vi "FGV Rezepte wechseln.vi"(0 "Rezepte":string, 1 "AK/man":T1, 5 "Rezeptindex":i32, 7 "Diesel":u16(ring) caption="Diesel:" items=["---"], 9 "Gasoline":u16(ring) caption="Gasoline:" items=["---"], 11 "error in (no error)":errorcluster caption="Fehler (Eingang, kein Fehler)", 12 "Natural Gas":u16(ring) caption="Natural Gas:" items=["---"], 13 "Aktion":T2) -> (3 "AK/man":T1, 4 "Rezepte":string[](array[string]), 6 "Rezeptindex":i32, 8 "Diesel":u16, 10 "Gasoline":u16, 14 "Natural Gas":u16, 15 "error out":errorcluster caption="Fehler (Ausgang)")   [LabVIEW 2020, in "FT-IR.lvlib"]
uses:
  FT-IR.lvlib
  Aktion FGV Rezepte wechseln.ctl
  AK-manuell.ctl
  Allgemein/allgemeine Sub-VIs.lvlib
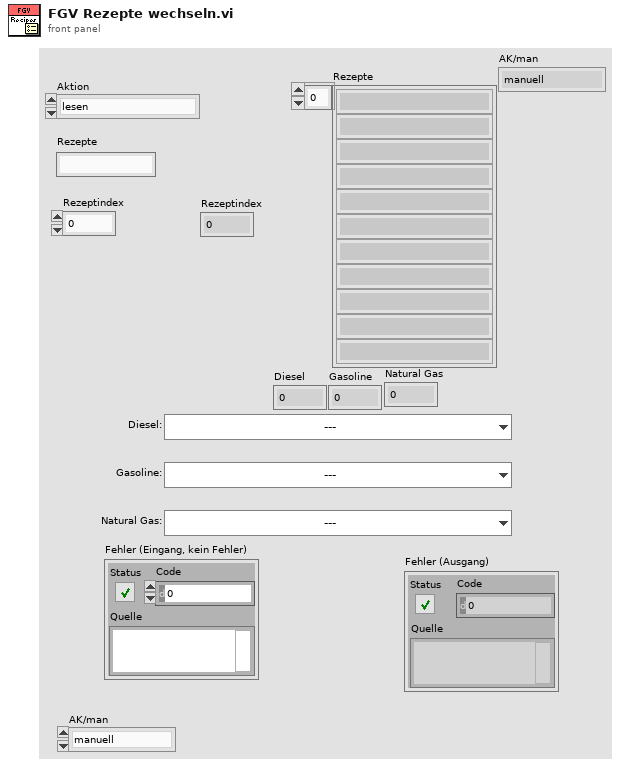
[diagram p1: front panel]
types:
  T1 = typedef "FT-IR.lvlib/AK-manuell.ctl" = enum16{"manuell", "Diesel", "CNG", "Gasoline"}
  T2 = typedef "FT-IR.lvlib/Aktion FGV Rezepte wechseln.ctl" = enum16{"lesen", "Rezepte", "Rezeptindex", "Diesel", "Gasoline", "NCG", "laden", "speichern", "AK/Man"}
  T3 = cluster{"Diesel":u16, "Gasoline":u16, "Natural Gas":u16}
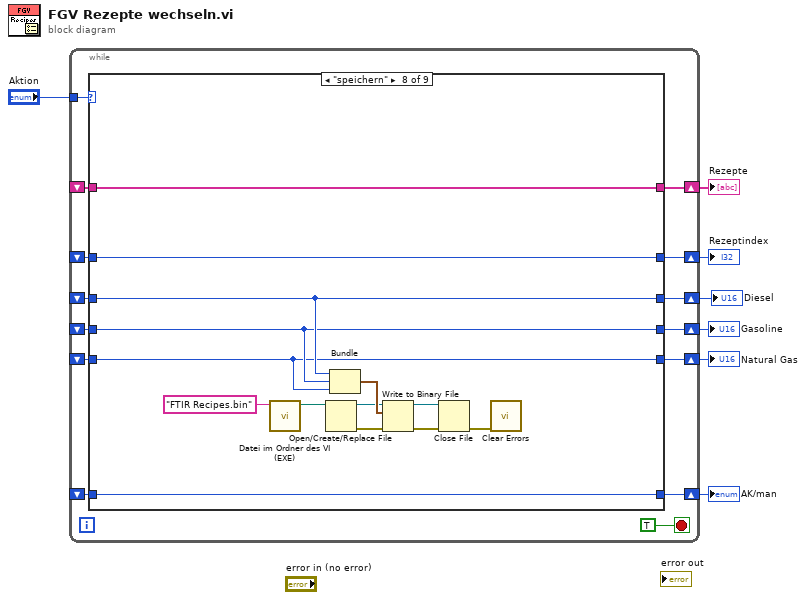
[diagram p0: block diagram]
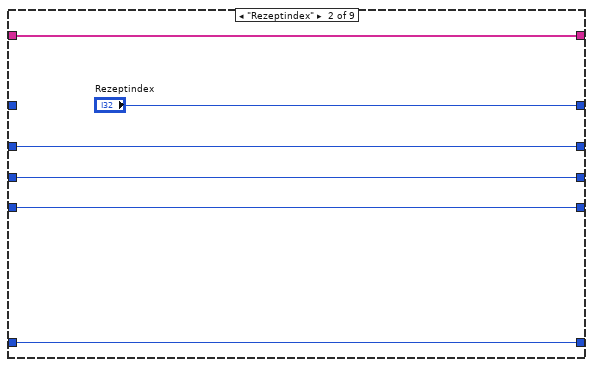
[diagram p3: hidden frame]
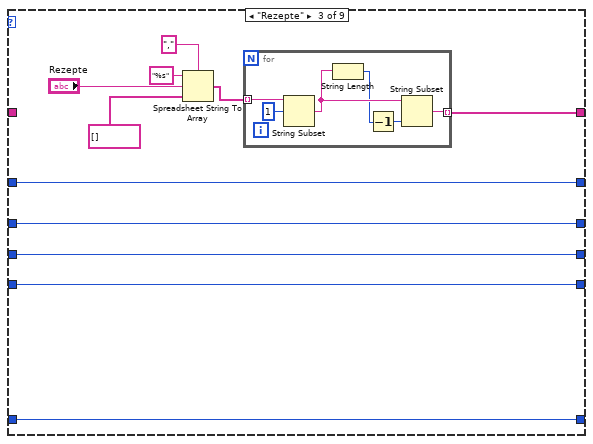
[diagram p4: hidden frame]
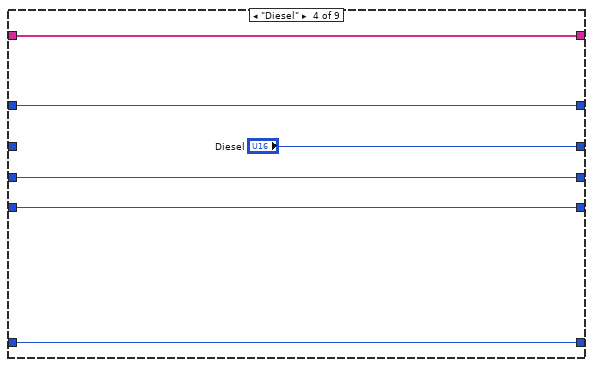
[diagram p5: hidden frame]
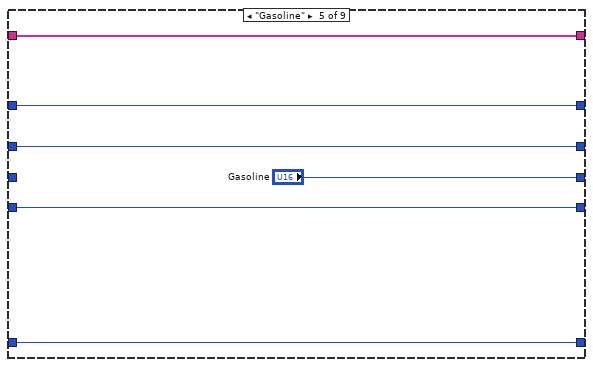
[diagram p6: hidden frame]
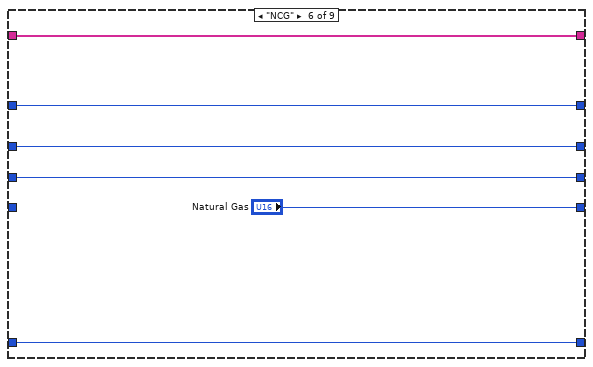
[diagram p7: hidden frame]
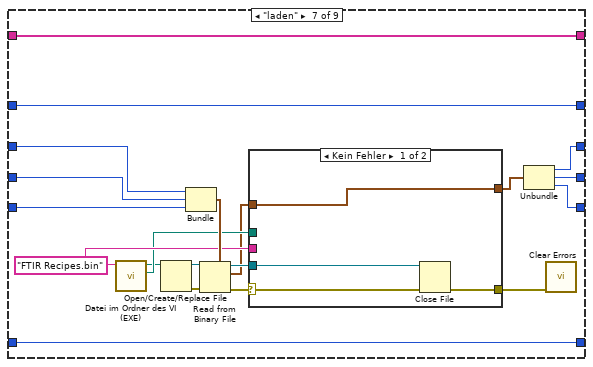
[diagram p8: hidden frame]
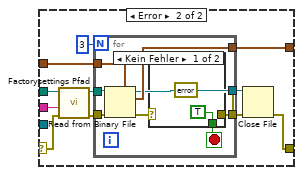
[diagram p9: hidden frame]
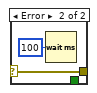
[diagram p10: hidden frame]
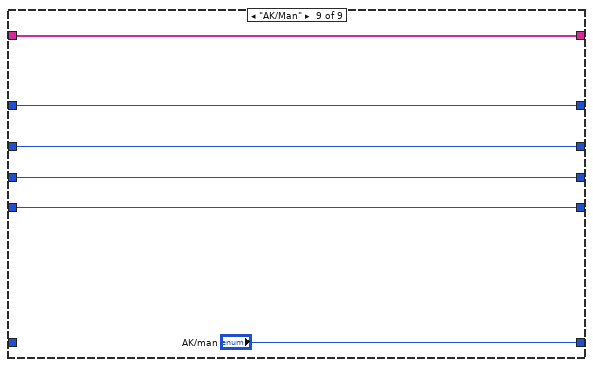
[diagram p11: hidden frame]
diagram:
  n1 = while {
    tunnel: "Aktion" -> [w20]
    shift-right: [w19] -> w6
    shift-left: _ -> [w18]
    shift-right: [w17] -> w5
    shift-left: _ -> [w16]
    shift-right: [w15] -> w4
    shift-left: _ -> [w14]
    shift-right: [w13] -> w3
    shift-left: _ -> [w12]
    shift-right: [w11] -> w2
    shift-left: _ -> [w10]
    shift-right: [w9] -> w1
    shift-left: _ -> [w8]
    stop <- TRUE stop-if-true
    n2 = case shown="\"speichern\"" w20 {
      tunnel: [w27 w33 w39 w56 w62 w68 w88 w129 w135] -> w19
      tunnel: w18 -> [w27 w33 _ w56 w62 w68 w88 w129 w135]
      tunnel: [w26 "Rezeptindex" w38 w55 w61 w67 w87 w128 w134] -> w17
      tunnel: w16 -> [w26 _ w38 w55 w61 w67 w87 w128 w134]
      tunnel: [w25 w31 w37 "Diesel" w60 w66 w82 w126 w133] -> w15
      tunnel: w14 -> [w25 w31 w37 _ w60 w66 w85 w126 w133]
      tunnel: [w24 w30 w36 w53 "Gasoline" w65 w81 w125 w132] -> w13
      tunnel: w12 -> [w24 w30 w36 w53 _ w65 w84 w125 w132]
      tunnel: [w23 w29 w35 w52 w58 "Natural Gas" w80 w124 w131] -> w11
      tunnel: w10 -> [w23 w29 w35 w52 w58 _ w83 w124 w131]
      tunnel: [w22 w28 w34 w51 w57 w63 w79 w122 "AK/man"] -> w9
      tunnel: w8 -> [w22 w28 w34 w51 w57 w63 w79 w122 _]
      frame "lesen", Default {
      }
      frame "Rezeptindex" {
      }
      frame "Rezepte" {
        n3 = Spreadsheet String To Array(delimiter (Tab)="," ("Trennzeichen (Tabulator)"), format string="%s" ("Format-String"), spreadsheet string="Rezepte", array type (2D Dbl)=string[] []) -> (array=w40:string[])
        n4 = for {
          tunnel: w40 -> [w50] mode=indexing
          tunnel: [w45] -> w39 mode=indexing
          n5 = String Subset(string=w50, offset (0)=1 ("Offset (0)")) -> (substring=w48:string)  [unwired: 1 in]
          n6 = String Length(string=w48) -> (length=w46:i32)
          n7 = Decrement(x=w46) -> (x-1=w47:i32)
          n8 = String Subset(string=w48, length (rest)=w47) -> (substring=w45:string)  [unwired: 1 in]
        }
      }
      frame "Diesel" {
      }
      frame "Gasoline" {
      }
      frame "NCG" {
      }
      frame "laden" {
        w76 = "FTIR Recipes.bin" ("Dateiname")
        n9 = call "Datei im Ordner des VI (EXE).vi"("Dateiname"=w76) -> ("Ordner des Haupt-VIs"=w75:path, "Dateipfad im Ordner des Haupt-VIs"=w69:path)  [unwired: 8 in, 1 out]
        n10 = Open/Create/Replace File(file path (use dialog)=w69) -> (refnum out=w70:refnum<file>, error out=w71:errorcluster)  [unwired: 5 in, 1 out]
        n11 = Bundle("Diesel"=w85, "Gasoline"=w84, "Natural Gas"=w83) -> (w86:T3)  [unwired: 1 in]
        n12 = Read from Binary File(5:w86, 8:w71, 11:w70) -> (0:w78:errorcluster, 2:w74:T3, 3:w77:refnum<file>)  [unwired: 4 out]
        n13 = case shown="Kein Fehler" w78 {
          selector: w78 -> [w91 w95]
          tunnel: w75 -> [_ w96]
          tunnel: w74 -> [w92 w94]
          tunnel: [w92 w102] -> w73
          tunnel: [w89 w100] -> w72
          tunnel: w77 -> [w90 _]
          tunnel: w76 -> [_ w93]
          frame No Error {
            n14 = Close File(refnum=w90, error in=w91) -> (error out=w89:errorcluster)  [unwired: 1 out]
          }
          frame Error {
            n15 = call "Factorysettings Pfad.vi"("error in (no error)"=w95, "Dateiname"=w93, "Ordner des Haupt-VIs"=w96) -> ("error out"=w97:errorcluster, "Pfad Factorysettings"=w98:path)  [unwired: 7 in]
            n16 = for {
              N: 3 -> [_]
              tunnel: w97 -> [w109]
              tunnel: w98 -> [w108]
              tunnel: [w107] -> w102
              tunnel: [w106] -> w101
              tunnel: [w105] -> w99
              tunnel: w94 -> [w104]
              stop <- w110 stop-if-true
              n17 = Read from Binary File(5:w104, 8:w109, 11:w108) -> (0:w111:errorcluster, 2:w107:T3, 3:w105:refnum<file>)  [unwired: 3 in, 1 out]
              n18 = case shown="Kein Fehler" w111 {
                selector: w111 -> [_ w114]
                tunnel: [TRUE _] -> w110
                tunnel: [errorcluster {"status"=FALSE, "code"=0, "source"=""} ("error IO") w114] -> w106
                frame No Error {
                }
                frame Error {
                  n19 = Wait (ms)(milliseconds to wait=u32 100 ("Zu wartende ms")) -> ()  [unwired: 1 out]
                }
              }
            }
            n20 = Close File(refnum=w99, error in=w101) -> (error out=w100:errorcluster)  [unwired: 1 out]
          }
        }
        n21 = Unbundle(w73) -> ("Diesel"=w82:u16, "Gasoline"=w81:u16, "Natural Gas"=w80:u16)
        n22 = call <vilib>:"Clear Errors.vi"("error in (no error)"=w72) -> ()  [unwired: 5 in, 2 out]
      }
      frame "speichern" {
        n23 = call "Datei im Ordner des VI (EXE).vi"("Dateiname"="FTIR Recipes.bin") -> ("Dateipfad im Ordner des Haupt-VIs"=w118:path)  [unwired: 8 in, 2 out]
        n24 = Open/Create/Replace File(file path (use dialog)=w118) -> (refnum out=w117:refnum<file>, error out=w116:errorcluster)  [unwired: 5 in, 1 out]
        n25 = Bundle("Diesel"=w126, "Gasoline"=w125, "Natural Gas"=w124) -> (w123:T3)  [unwired: 1 in]
        n26 = Write to Binary File(file (use dialog)=w117, data=w123, error in=w116) -> (refnum out=w120:refnum<file>, error out=w121:errorcluster)  [unwired: 3 in, 1 out]
        n27 = Close File(refnum=w120, error in=w121) -> (error out=w119:errorcluster)  [unwired: 1 out]
        n28 = call <vilib>:"Clear Errors.vi"("error in (no error)"=w119) -> ()  [unwired: 5 in, 2 out]
      }
      frame "AK/Man" {
      }
    }
  }
  "Rezepte" <- w6
  "Rezeptindex" <- w5
  "Diesel" <- w4
  "Gasoline" <- w3
  "Natural Gas" <- w2
  "AK/man" <- w1
